vi "Write Configuration File.vi"(8 "error in (no error)":errorcluster, 11 "Instrument.Lockin":refnum<class "Instrument.Lockin.lvclass">) -> (0 "error out":errorcluster, 3 "Instrument.Lockin out":refnum<class "Instrument.Lockin.lvclass">)   [LabVIEW 2019, in "Instrument.Lockin.lvclass"]
uses:
  Instrument.Lockin.lvclass
  C:/Program Files (x86)/National Instruments/LabVIEW 2019/user.lib/LevyLab/Instrument Framework/Instrument/Instrument.lvclass
  <userlib>/LevyLab/Instrument Framework/Instrument/Instrument.lvclass/Instrument.ctl
  <userlib>/LevyLab/Configuration/Configuration.lvclass/Configuration.ctl
  Instrument.Lockin.lvclass/Instrument.Lockin.ctl
  <userlib>/LevyLab/Configuration/Write Section.vi
  <userlib>/LevyLab/Instrument Framework/Instrument/Instrument.lvclass
  C:/Program Files (x86)/National Instruments/LabVIEW 2019/vi.lib/JKI/JKI SMO/SMO/SMO.lvclass
  <vilib>/JKI/JKI SMO/SMO/Protected/ThisLevelClassName.vi
  <userlib>/LevyLab/Instrument Framework/Instrument Types/Lockin/Instrument.LockinAPI.lvclass
  <userlib>/LevyLab/Configuration/Configuration.lvclass
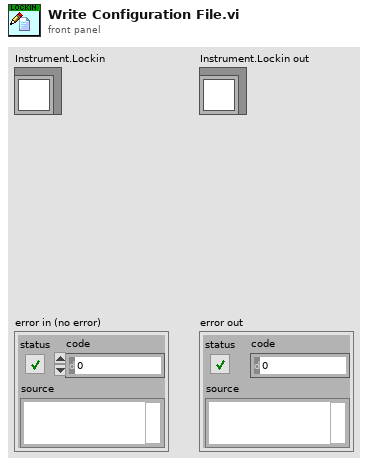
[diagram p1: front panel]
types:
  T1 = typedef "Instrument.DAQ.lvclass/Configuration--Cluster.ctl" = cluster{"DAQ":T2, "Channels":T18, "Prefilter":T26, "Offset and Gain":T27, "Limit Amplitude":T30, "Link Frequencies":T31, "Sweep":T32}
  T2 = typedef "Instrument.DAQ.lvclass/Configuration.DAQ--Cluster.ctl" = cluster{"Sampling":T3, "Simulation mode":T7, "AI":T8, "AO":T13, "Calibration":T16}
  T3 = typedef "Instrument.DAQ.lvclass/DAQ.Sampling--Cluster.ctl" = cluster{"Sampling":T4, "Sample Mode":T5, "Fs Mode":T6, "Fs Multiplier":dbl, "Refresh Rate (Hz)":dbl, "Decimation.PreDSP":i32, "Decimation.PostDSP":i32, "Fs.Output":dbl}
  T4 = typedef "Instrument.DAQ.lvclass/DAQ.Sampling.Sampling--Cluster.ctl" = cluster{"Fs":dbl, "#s":i32}
  T5 = typedef "Instrument.DAQ.lvclass/DAQ.Sampling.Sample Mode--Ring.ctl" = i32
  T6 = typedef "Instrument.DAQ.lvclass/DAQ.Sampling.Fs Mode--enum.ctl" = enum16{"Manual", "Auto Fs", "Max Fs"}
  T7 = typedef "Instrument.DAQ.lvclass/Simulation Mode--enum.ctl" = enum16{"AI = HW simulated", "AI = noise*AO", "AI = waveguide"}
  T8 = typedef "Instrument.DAQ.lvclass/DAQ.Config.AI--Cluster--Array.ctl" = T9[]
  T9 = typedef "Instrument.DAQ.lvclass/DAQ.Config.AI--Cluster.ctl" = cluster{"Channels":tag, "Coupling":T10, "Range":T11, "input terminal configuration":i32, "Type":T12}
  T10 = typedef "Instrument.DAQ.lvclass/DAQ.Config.AI.Coupling--enum.ctl" = u16
  T11 = typedef "Instrument.DAQ.lvclass/DAQ.Config.AI.Range--enum.ctl" = enum16{"±0.316", "±1.00", "±3.16", "±10.0", "±31.6", "±42.4"}
  T12 = typedef "Instrument.DAQ.lvclass/DAQ.Type--enum.ctl" = enum16{"None", "USB-4431", "PXI-446x"}
  T13 = typedef "Instrument.DAQ.lvclass/DAQ.Config.AO--Cluster--Array.ctl" = T14[]
  T14 = typedef "Instrument.DAQ.lvclass/DAQ.Config.AO--Cluster.ctl" = cluster{"Channels":tag, "Range":T15, "output terminal configuration":i32, "Type":T12}
  T15 = typedef "Instrument.DAQ.lvclass/DAQ.Config.AO.Range--enum.ctl" = enum16{"±0.1", "±1.0", "±10.0"}
  T16 = typedef "Instrument.DAQ.lvclass/DAQ.Calibration--Cluster--Array.ctl" = T17[]
  T17 = typedef "Instrument.DAQ.lvclass/DAQ.Calibration--Cluster.ctl" = cluster{"Active Device":string, "SelfCal.LastDate/Time":dbl, "SelfCal.LastTemp":dbl, "DevTemp":dbl, "calibration due?":bool}
  T18 = typedef "Instrument.DAQ.lvclass/Configuration.Channels--Cluster.ctl" = cluster{"Cfg_AO":T19, "Cfg_AI":T22, "Cfg_REF":T24}
  T19 = typedef "Instrument.DAQ.lvclass/AO.Channel--Cluster--Array.ctl" = T20[]
  T20 = typedef "Instrument.DAQ.lvclass/AO.Channel--Cluster.ctl" = cluster{"Enable?":bool, "Channel":i32, "Amplitude":dbl, "Offset":dbl, "Frequency":dbl, "Phase":dbl, "Function":T21, "Sweeping?":bool}
  T21 = typedef "Instrument.DAQ.lvclass/AO.Channel.Function--Enum.ctl" = enum16{"Sine", "Triangle", "Square"}
  T22 = typedef "Instrument.DAQ.lvclass/AI.Channel--Cluster--Array.ctl" = T23[]
  T23 = typedef "Instrument.DAQ.lvclass/AI.Channel--Cluster.ctl" = cluster{"Enable?":bool, "Channel":i32, "References":i32[]}
  T24 = typedef "Instrument.DAQ.lvclass/REF.Channel--Cluster--Array.ctl" = T25[]
  T25 = typedef "Instrument.DAQ.lvclass/REF.Channel--Cluster.ctl" = cluster{"Enable?":bool, "Channel":i32, "Frequency":dbl, "Phase":dbl, "TC":dbl, "Roll-Off":i32}
  T26 = typedef "Instrument.DAQ.lvclass/Configuration.Prefilter--Cluster.ctl" = cluster{"60 Hz":bool, "Low Pass":bool, "Low Pass Cutoff (Hz)":dbl}
  T27 = typedef "Instrument.DAQ.lvclass/Channel.GainsAndOffsets--Cluster.ctl" = cluster{"Offset_AI":T28, "Gain_AI":T28, "Gain_AO":T28}
  T28 = typedef "Instrument.DAQ.lvclass/Channel.Gain--Cluster--Array.ctl" = T29[]
  T29 = typedef "Instrument.DAQ.lvclass/Channel.Gain--Cluster.ctl" = cluster{"Channel":string, "Gain":dbl}
  T30 = typedef "Instrument.DAQ.lvclass/Configuration.LimitAmplitude--Cluster.ctl" = cluster{"Limit?":bool, "Limit (V)":dbl}
  T31 = typedef "Instrument.DAQ.lvclass/Configuration.LinkFrequencies--Cluster.ctl" = cluster{"Link?":bool, "Frequency (Hz)":dbl}
  T32 = typedef "Instrument.DAQ.lvclass/Sweep.Configuration--Cluster.ctl" = cluster{"Sweep Time (s)":dbl, "Initial Wait (s)":dbl, "Return to Start":bool, "Channels":T33}
  T33 = typedef "Instrument.DAQ.lvclass/Sweep.Channel--Cluster--Array.ctl" = T34[]
  T34 = typedef "Instrument.DAQ.lvclass/Sweep.Channel--Cluster.ctl" = cluster{"Enable?":bool, "Channel":u16, "Start":dbl, "End":dbl, "Pattern":T35, "Table":dbl[]}
  T35 = typedef "Instrument.DAQ.lvclass/Sweep.Pattern--Enum.ctl" = enum16{"Ramp /", "Ramp /\\", "Smooth Ramp _/", "Smooth Ramp _/\\_", "Table"}
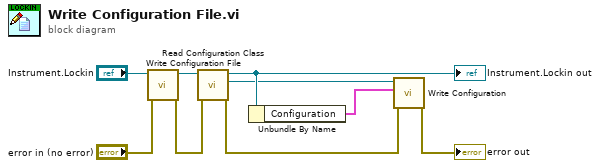
[diagram p0: block diagram]
diagram:
  n1 = call-parent "Write Configuration File.vi"("error in (no error)"="error in (no error)", "Instrument in"="Instrument.Lockin") -> ("error out"=w6:errorcluster, "Instrument out"=w4:refnum<class "Instrument.Lockin.lvclass">)  [unwired: 8 in]
  n2 = call <userlib>:"Read Configuration Class.vi"("error in (no error)"=w6, "Instrument in"=w4) -> ("error out"=w2:errorcluster, "Configuration"=w1:refnum<class "Configuration.lvclass">, "Instrument out"=w3:refnum<class "Instrument.Lockin.lvclass">)  [unwired: 7 in]
  "Instrument.Lockin out" <- w3
  n3 = Unbundle By Name(w3) -> ("Configuration"=w8:T1)
  n4 = call <userlib>:"Write Configuration.vi"("error in (no error)"=w2, "Variant"=w8, "Configuration in"=w1) -> ("error out"=→"error out":errorcluster)  [unwired: 7 in, 1 out]
